vi "Write Impulse Positions.vi"(8 "error in (no error)":errorcluster, 10 "Impulse Positions":T2(array[cluster]), 11 "Abstract Fit in":refnum<class "Abstract Fit.lvclass">) -> (0 "error out":errorcluster, 3 "Abstract Fit out":refnum<class "Abstract Fit.lvclass">)   [LabVIEW 2016, in "Abstract Fit.lvclass"]
uses:
  Abstract Fit.lvclass
  type-defs/TD_Impulse Planes.ctl
  Abstract Fit.lvclass/Abstract Fit.ctl
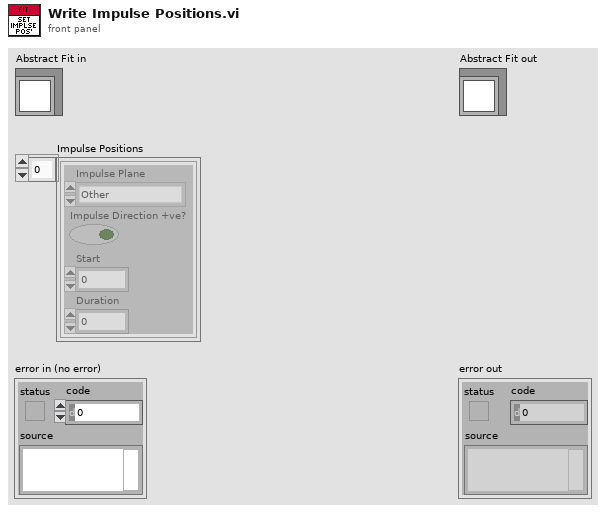
[diagram p1: front panel]
types:
  T1 = typedef "TD_Impulse Planes.ctl" = enum16{"Other", "Yaw", "Pitch", "Roll", "LARP", "RALP"}
  T2 = cluster{"Impulse Plane":T1, "Impulse Direction +ve?":bool, "Start":i32, "Duration":i32}[]
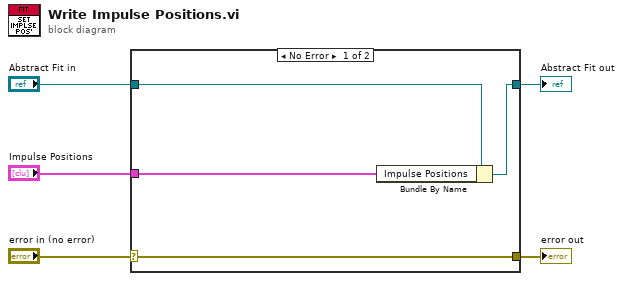
[diagram p0: block diagram]
diagram:
  n1 = case shown="No Error" "error in (no error)" {
    selector: "error in (no error)" -> [w9 w10]
    tunnel: [w9 w10] -> w4
    tunnel: [w7 w11] -> w2
    tunnel: "Abstract Fit in" -> [w8 w11]
    tunnel: "Impulse Positions" -> [w6 _]
    frame No Error {
      n2 = Bundle By Name(cluster=w8, "Impulse Positions"=w6) -> (w7:refnum<class "Abstract Fit.lvclass">)
    }
    frame Error {
    }
  }
  "error out" <- w4
  "Abstract Fit out" <- w2
